vi "filter targets.vi"(10 "targets to load":string[](array[string]), 11 "targets in":T1[](array[typedef])) -> (3 "targets out":T1[](array[typedef]))   [LabVIEW 2013, in "PLConfigurationSerializer.lvlib"]
doc: "Filters a list of targets down to just the targets desired to load."
uses:
  PLConfigurationSerializer.lvlib
  targetlist.ctl
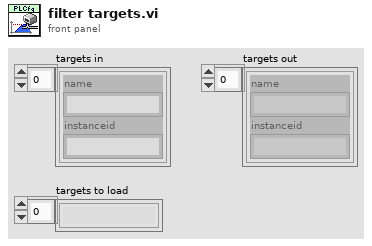
[diagram p1: front panel]
types:
  T1 = typedef "PLConfigurationSerializer.lvlib/targetlist.ctl" = cluster{"name":string, "instanceid":string}
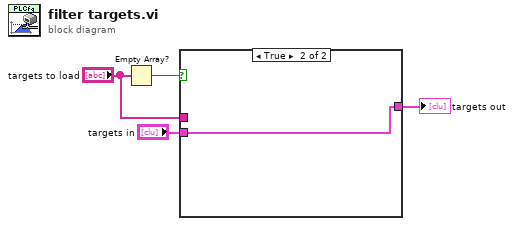
[diagram p0: block diagram]
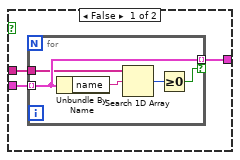
[diagram p2: hidden frame]
diagram:
  n1 = Empty Array?(array="targets to load") -> (empty?=w4:bool)
  n2 = case shown="True" w4 {
    tunnel: [w6 w13] -> w3
    tunnel: "targets in" -> [w7 w13]
    tunnel: "targets to load" -> [w5 _]
    frame False {
      n3 = for {
        tunnel: w7 -> [w12] mode=indexing
        tunnel: [w12] -> w6 mode=indexing if=w8
        tunnel: w5 -> [w11]
        n4 = Unbundle By Name(w12) -> ("name"=w10:string)
        n5 = Search 1D Array(1D array=w11, element=w10) -> (index of element=w9:i32)  [unwired: 1 in]
        n6 = Greater Or Equal To 0?(x=w9) -> (x >= 0?=w8:bool)
      }
    }
    frame True {
    }
  }
  "targets out" <- w3
